vi "Main.vi"() -> ()   [LabVIEW 2020]
uses:
  controls/sliding_panel_left.ctl
  controls/power_chart.ctl
  controls/max_power_slider.ctl
  controls/tiny_map_icon_basic.ctl
  controls/sliding_panel_right.ctl
  controls/wind_chart.ctl
  controls/sliding_panel_console.ctl
  controls/day_of_month_slider.ctl
  controls/single_multicity_basic.ctl
  controls/plus_basic.ctl
  controls/minus_basic.ctl
  controls/wind_turbine_icon_basic.ctl
  controls/tiny_plots_icon_basic.ctl
  <vilib>/Platform/TimedLoop/XDataNode/timing_clust.ctl
  <vilib>/Platform/TimedLoop/XDataNode/nitl_modes.ctl
  <vilib>/Platform/TimedLoop/XDataNode/wakeup.ctl
  <vilib>/Platform/TimedLoop/XDataNode/XDataNode.xnode
  <vilib>/Platform/TimedLoop/XDataNode/XDNodeRunTimeDep.lvlib
panel:
  in  "show_map":T1
  in  "show_plots":T2
  in  "sliding_panel_console":T3={"Days of Month"=29, "multicity"=FALSE, "plus"=FALSE, "minus"=FALSE} {"Days of Month" min=1 max=30 step=1 scale=0.0..30.0}
  out "sliding_panel_right":T8={"title"="Select a city", "Wind"=[]}
  out "sliding_panel_left":T10={"title"="Power Statistics", "Power"=[], "max_power_slide"=3.1127450980392157, "max_power_digi"=0.13, "max_power_title"="Select a city (# days)"} {"max_power_digi" format="%#_3g"; "max_power_slide" scale=0.0..40.0}
  out "signature":string="Thoric 2011"
  out "title":string="Select a city"
  in  "USA":T13 caption="Texas (USA)"
  in  "costa_rica":T13 caption="Puerto Limon (Costa Rica)"
  in  "brazil":T13 caption="Brasilia (Brazil)"
  in  "south_africa":T13 caption="Cape Good Hope (South Africa)"
  in  "australia":T13 caption="Marrara (Australia)"
  in  "japan":T13 caption="Ise Bay (Japan)"
  in  "india":T13 caption="Mumbai (India)"
  in  "israel":T13 caption="Sde-Dov (Israel)"
  in  "germany":T13 caption="Berlin (Germany)"
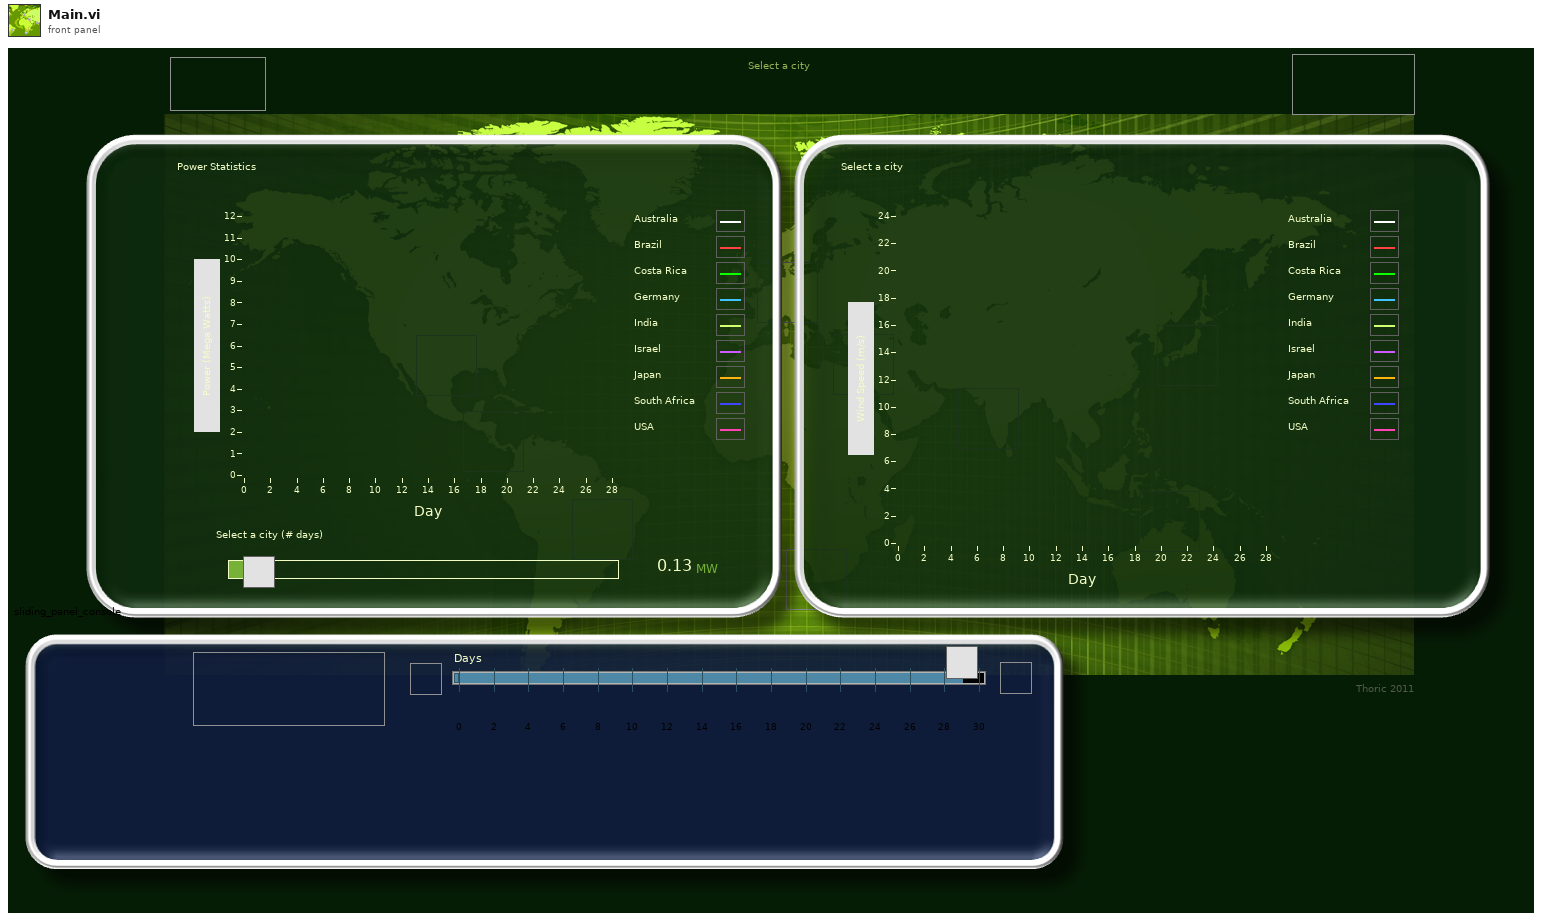
[diagram p1: front panel]
types:
  T1 = typedef "tiny_map_icon_basic.ctl" = bool
  T2 = typedef "tiny_plots_icon_basic.ctl" = bool
  T3 = typedef "sliding_panel_console.ctl" = cluster{"Days of Month":T4, "multicity":T5, "plus":T6, "minus":T7}
  T4 = typedef "day_of_month_slider.ctl" = i32
  T5 = typedef "single_multicity_basic.ctl" = bool
  T6 = typedef "plus_basic.ctl" = bool
  T7 = typedef "minus_basic.ctl" = bool
  T8 = typedef "sliding_panel_right.ctl" = cluster{"title":string, "Wind":T9}
  T9 = typedef "wind_chart.ctl" = dbl[][]
  T10 = typedef "sliding_panel_left.ctl" = cluster{"title":string, "Power":T11, "max_power_slide":T12, "max_power_digi":dbl, "max_power_title":string}
  T11 = typedef "power_chart.ctl" = dbl[][]
  T12 = typedef "max_power_slider.ctl" = dbl
  T13 = typedef "wind_turbine_icon_basic.ctl" = bool
  T14 = enum8{"Enabled", "Disabled", "Disabled and Grayed Out"}
  T15 = typedef "XDNodeRunTimeDep.lvlib/timing_clust.ctl" = cluster{"Expected End [f-1]":u64, "Actual End [f-1]":u64, "Finished Late? [f-1]":bool, "Expected End [i-1]":u64, "Actual End [i-1]":u64, "Finished Late? [i-1]":bool, "Expected Start [i]":u64, "Actual Start [i]":u64, "Expected Start [f]":u64, "Actual Start [f]":u64, "Source Name":string, "Structure Name":string, "Period":i64, "Deadline":i64, "Offset":i64, "Start":i64, "Priority":i32, "Timeout":i32, "Mode":T16, "Wakeup Reason":T17, "Error":errorcluster, "Source Type":string, "Secondary Source Type":string, "Global End Time":u64, "Global Start Time":u64, "Frame Duration":u64, "Iteration Duration":u64, "Assigned CPU":i32, "I/O Scan Engine Mode":u32}
  T16 = typedef "XDNodeRunTimeDep.lvlib/nitl_modes.ctl" = enum32{"No Change", "Process missed periods, maintain original phase", "Discard missed periods, maintain original phase", "Process missed periods, ignore original phase", "Discard missed periods, ignore original phase"}
  T17 = typedef "XDNodeRunTimeDep.lvlib/wakeup.ctl" = enum32{"Normal", "Aborted", "Asynchronous wakeup", "Timing source error", "Timed loop error", "Timeout"}
  T18 = enum32{"invalid app kind", "Development System", "Run Time System", "Student Edition", "Embedded LabVIEW", "Evaluation", "Custom"}
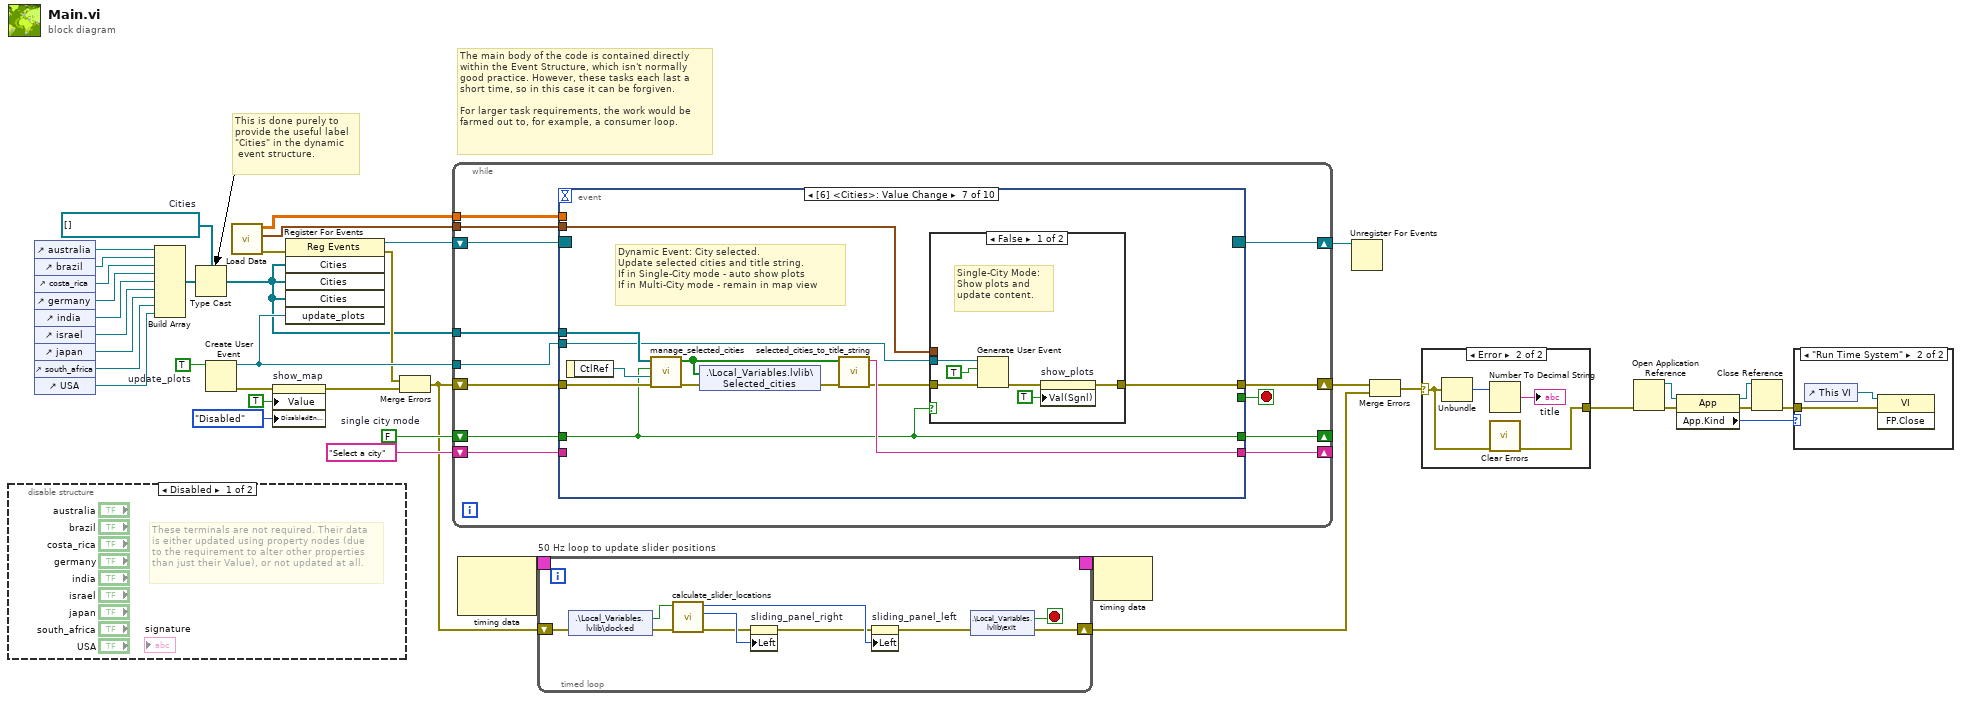
[diagram p0: block diagram]
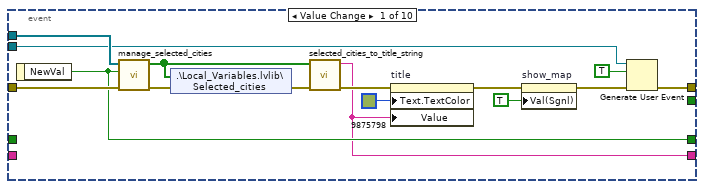
[diagram p5: hidden frame]
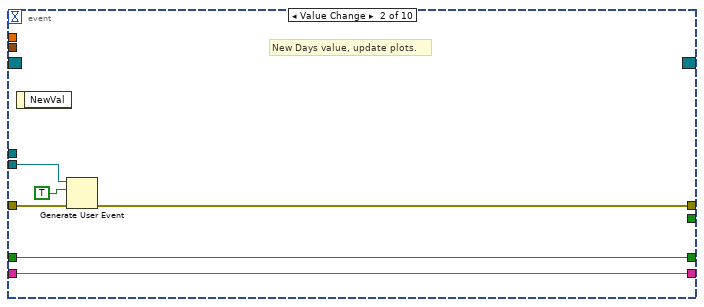
[diagram p6: hidden frame]
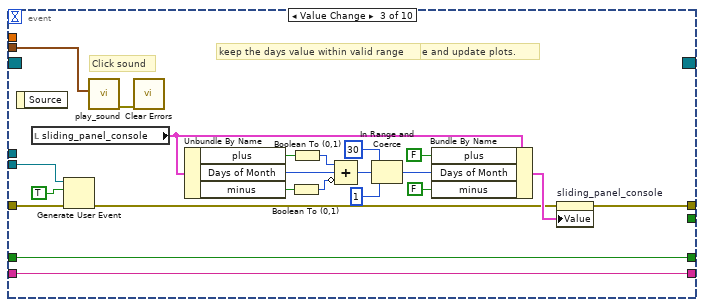
[diagram p7: hidden frame]
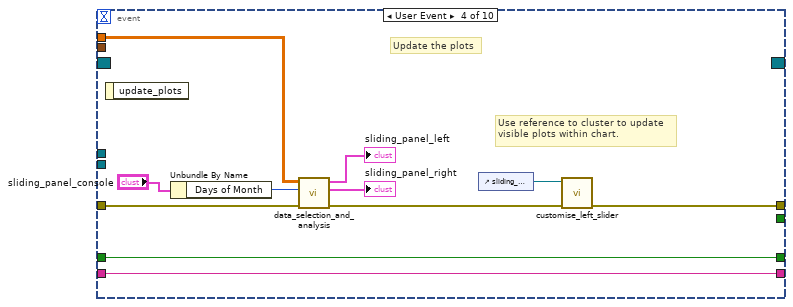
[diagram p8: hidden frame]
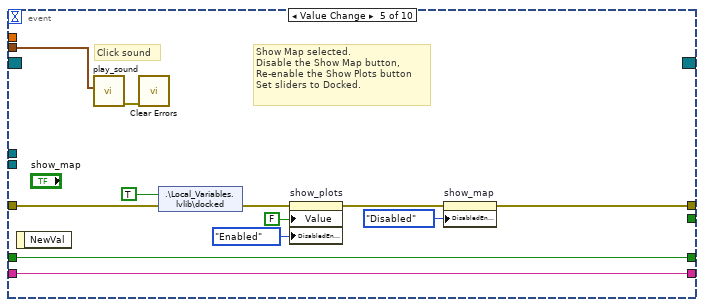
[diagram p9: hidden frame]
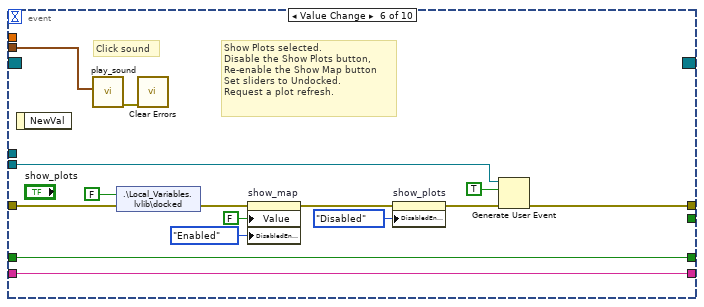
[diagram p10: hidden frame]
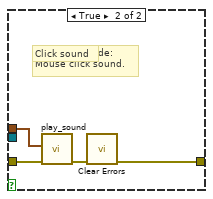
[diagram p11: hidden frame]
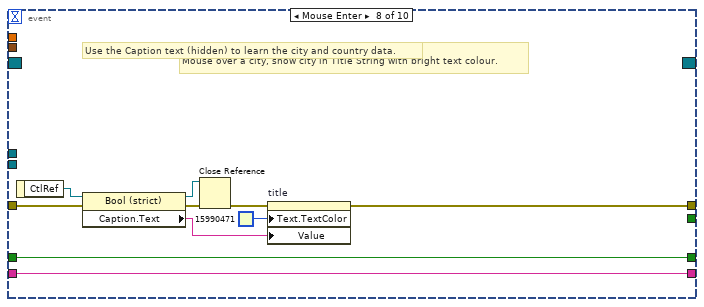
[diagram p12: hidden frame]
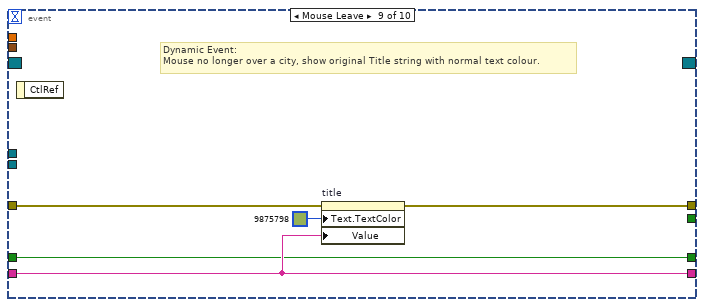
[diagram p13: hidden frame]
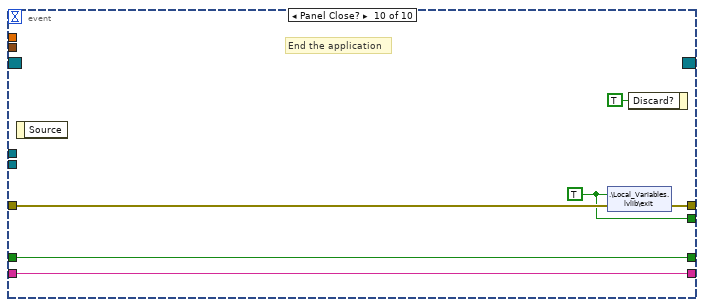
[diagram p14: hidden frame]
diagram:
  w12 = refnum<vi>[] []  # Cities
  w22 = T5 FALSE  # single city mode
  w25 = TRUE  # update_plots
  # "The main body of the code is contained directly\nwithin the Event Structure, which isn't normally\ngood practice. However, these tasks each last a\nshort time, so in this case it can be forgiven.\n\nFor larger task requirements, the work would be\nfarmed out to, for example, a consumer loop."
  # "This is done purely to\nprovide the useful label\n\"Cities\" in the dynamic\n event structure."
  n1 = disable-structure shown="Disabled" {
    frame Disabled {
      # "These terminals are not required. Their data\nis either updated using property nodes (due\nto the requirement to alter other properties\nthan just their Value), or not updated at all."
    }
    frame Enabled {
    }
  }
  n2 = control-ref of="australia"() -> (w36:refnum<vi>)
  n3 = control-ref of="brazil"() -> (w35:refnum<vi>)
  n4 = control-ref of="costa_rica"() -> (w34:refnum<vi>)
  n5 = control-ref of="germany"() -> (w33:refnum<vi>)
  n6 = control-ref of="india"() -> (w32:refnum<vi>)
  n7 = control-ref of="israel"() -> (w31:refnum<vi>)
  n8 = control-ref of="japan"() -> (w30:refnum<vi>)
  n9 = control-ref of="south_africa"() -> (w29:refnum<vi>)
  n10 = control-ref of="USA"() -> (w28:refnum<vi>)
  n11 = Build Array(w36, w35, w34, w33, w32, w31, w30, w29, w28) -> (w14:refnum<vi>[])
  n12 = Type Cast(type=w12, x=w14) -> (*(type *) &x=w13:refnum<vi>[])
  n13 = Create User Event(user event datatype=w25) -> (user event=w24:refnum<user-event>, error out=w9:errorcluster)  [unwired: 1 in]
  n14 = call "Load Data.vi"() -> ("error out"=w20:errorcluster, "Sound WAV data"=w21:waveform(dbl)[], "Wind Data"=w23:dbl[][])  [unwired: 9 in]
  n15 = property on="show_map" class="Bool (strict)"(error in=w9, "Value"=TRUE, "DisabledEnum"=T14."Disabled" ("Disabled")) -> (error out=w8:errorcluster)  [unwired: 1 in, 1 out]
  n16 = register-events(error in=w20, w13, w13, w13, w24) -> (reference out=w37:refnum<event-registration>, error out=w19:errorcluster)  [unwired: 1 in]
  n17 = Merge Errors(w19, w8) -> (w18:errorcluster)
  n18 = while {
    shift-right: [w51] -> w17
    shift-left: w18 -> [w52]
    shift-right: [w48] -> w27
    shift-left: w37 -> [w49]
    shift-right: [w46] -> _
    shift-left: "Select a city" ("title") -> [w47]
    shift-right: [w44] -> _
    shift-left: w22 -> [w45]
    tunnel: w13 -> [w43]
    tunnel: w24 -> [w42]
    tunnel: w23 -> [w41]
    tunnel: w21 -> [w40]
    stop <- w50 stop-if-true
    n19 = event shown="[6] <Cities>: Value Change" {
      selector: w49 -> [_ _ _ _ _ _ _ _ _ _]
      dyn-events: [_ _ _ _ _ _ _ _ _ _] -> w48
      timeout: _ -> [_ _ _ _ _ _ _ _ _ _]
      tunnel: w52 -> [w67 w70 w81 w104 w116 w131 w141 w159 w169 w175]
      tunnel: [w55 w68 w93 w96 w110 w128 w136 w163 w168 w176] -> w51
      tunnel: [_ _ _ _ _ _ _ _ _ w174] -> w50
      tunnel: w47 -> [_ w73 w95 w106 w118 w133 _ w164 w167 w172]
      tunnel: [w59 w73 w95 w106 w118 w133 w144 w164 w167 w172] -> w46
      tunnel: w45 -> [_ w72 w94 w105 w117 w132 w138 w160 w166 w171]
      tunnel: [w66 w72 w94 w105 w117 w132 w138 w160 w166 w171] -> w44
      tunnel: w43 -> [w65 _ _ _ _ _ w143 _ _ _]
      tunnel: w42 -> [w54 w69 w79 _ _ w124 w134 _ _ _]
      tunnel: w41 -> [_ _ _ w103 _ _ _ _ _ _]
      tunnel: w40 -> [_ _ w74 _ w107 w119 w135 _ _ _]
      event Value Change {
        n20 = event-data() -> ("NewVal"=w66:T5)  [unwired: 1 in]
        n21 = call "manage_selected_cities.vi"("error in"=w67, "multicity"=w66, "Selected_cities_refs[]"=w65) -> ("error out"=w64:errorcluster, "Selected_Cities[]"=w62:T13[])  [unwired: 7 in]
        n22 = shared-variable ".\\Local_Variables.lvlib\\Selected_cities"(w62, error in=w64) -> (error out=w63:errorcluster)
        n23 = call "selected_cities_to_title_string.vi"("error in"=w63, "selected_cities"=w62) -> ("error out"=w60:errorcluster, "title_string"=w59:string)  [unwired: 8 in]
        n24 = property on="title" class="Str"(error in=w60, "Text.TextColor"=u32 9875798, "Value"=w59) -> (error out=w58:errorcluster)  [unwired: 1 in, 1 out]
        n25 = property on="show_map" class="Bool (strict)"(error in=w58, "Val(Sgnl)"=TRUE ("docked")) -> (error out=w56:errorcluster)  [unwired: 1 in, 1 out]
        n26 = Generate User Event(user event=w54, event data cluster=TRUE ("event data"), error in=w56) -> (error out=w55:errorcluster)  [unwired: 1 in, 1 out]
      }
      event Value Change {
        # "New Days value, update plots."
        n27 = event-data() -> ()  [unwired: 1 in, 1 out]
        n28 = Generate User Event(user event=w69, event data cluster=TRUE ("event data"), error in=w70) -> (error out=w68:errorcluster)  [unwired: 1 in, 1 out]
      }
      event Value Change {
        # "keep the days value within valid range"
        # "Days +, Days - selected. Update Days value and update plots."
        # "Click sound"
        n29 = event-data() -> ()  [unwired: 1 in, 1 out]
        n30 = local read "sliding_panel_console"() -> (w92:T3)
        n31 = Generate User Event(user event=w79, event data cluster=TRUE ("event data"), error in=w81) -> (error out=w80:errorcluster)  [unwired: 1 in, 1 out]
        n32 = call "play_sound.vi"("Data"=w74) -> ("error out"=w75:errorcluster)  [unwired: 9 in]
        n33 = call <vilib>:"Clear Errors.vi"("error in (no error)"=w75) -> ()  [unwired: 5 in, 2 out]
        n34 = Unbundle By Name(w92) -> ("plus"=w88:T6, "Days of Month"=w89:T4, "minus"=w86:T7)
        n35 = Boolean To (0,1)(Boolean=w86) -> (0, 1=w85:i16)
        n36 = Boolean To (0,1)(Boolean=w88) -> (0, 1=w87:i16)
        n37 = Compound Arithmetic op=ADD(w87, w89, invert w85) -> (w90:T4)
        n38 = In Range and Coerce(upper limit=T4 30, x=w90, lower limit=T4 1) -> (coerced(x)=w78:T4)  [unwired: 1 out]
        n39 = Bundle By Name(cluster=w92, "plus"=T6 FALSE, "Days of Month"=w78, "minus"=T7 FALSE) -> (w91:T3)
        n40 = property on="sliding_panel_console" class="Clust (strict)"(error in=w80, "Value"=w91) -> (error out=w93:errorcluster)  [unwired: 1 in, 1 out]
      }
      event User Event {
        # "Use reference to cluster to update\nvisible plots within chart."
        # "Update the plots"
        n41 = event-data() -> ()  [unwired: 1 in, 1 out]
        n42 = Unbundle By Name("sliding_panel_console") -> ("Days of Month"=w101:T4)
        n43 = call "data_selection_and_analysis.vi"("error in"=w104, "days"=w101, "wind data in"=w103) -> ("error out"=w97:errorcluster, "sliding_panel_right"=→"sliding_panel_right":T8, "left_pane_cluster"=→"sliding_panel_left":T10)  [unwired: 6 in]
        n44 = control-ref of="sliding_panel_left"() -> (w98:refnum<vi>)
        n45 = call "customise_left_slider.vi"("error in"=w97, "slide_left_ref"=w98) -> ("error out"=w96:errorcluster)  [unwired: 9 in]
      }
      event Value Change {
        # "Show Map selected.\nDisable the Show Map button,\nRe-enable the Show Plots button\nSet sliders to Docked."
        # "Click sound"
        n46 = event-data() -> ()  [unwired: 1 in, 1 out]
        n47 = call "play_sound.vi"("Data"=w107) -> ("error out"=w108:errorcluster)  [unwired: 9 in]
        n48 = call <vilib>:"Clear Errors.vi"("error in (no error)"=w108) -> ()  [unwired: 5 in, 2 out]
        n49 = shared-variable ".\\Local_Variables.lvlib\\docked"(TRUE, error in=w116) -> (error out=w114:errorcluster)
        n50 = property on="show_plots" class="Bool (strict)"(error in=w114, "Value"=FALSE ("hide_map"), "DisabledEnum"=T14."Enabled" ("Disabled")) -> (error out=w111:errorcluster)  [unwired: 1 in, 1 out]
        n51 = property on="show_map" class="Bool (strict)"(error in=w111, "DisabledEnum"=T14."Disabled" ("Disabled")) -> (error out=w110:errorcluster)  [unwired: 1 in, 1 out]
      }
      event Value Change {
        # "Show Plots selected.\nDisable the Show Plots button,\nRe-enable the Show Map button\nSet sliders to Undocked.\nRequest a plot refresh."
        # "Click sound"
        n52 = event-data() -> ()  [unwired: 1 in, 1 out]
        n53 = call "play_sound.vi"("Data"=w119) -> ("error out"=w120:errorcluster)  [unwired: 9 in]
        n54 = shared-variable ".\\Local_Variables.lvlib\\docked"(FALSE, error in=w131) -> (error out=w127:errorcluster)
        n55 = call <vilib>:"Clear Errors.vi"("error in (no error)"=w120) -> ()  [unwired: 5 in, 2 out]
        n56 = property on="show_map" class="Bool (strict)"(error in=w127, "Value"=FALSE, "DisabledEnum"=T14."Enabled" ("Disabled")) -> (error out=w123:errorcluster)  [unwired: 1 in, 1 out]
        n57 = property on="show_plots" class="Bool (strict)"(error in=w123, "DisabledEnum"=T14."Disabled" ("Disabled")) -> (error out=w122:errorcluster)  [unwired: 1 in, 1 out]
        n58 = Generate User Event(user event=w124, event data cluster=TRUE ("event data"), error in=w122) -> (error out=w128:errorcluster)  [unwired: 1 in, 1 out]
      }
      event Value Change {
        # "Dynamic Event: City selected.\nUpdate selected cities and title string.\nIf in Single-City mode - auto show plots\nIf in Multi-City mode - remain in map view"
        n59 = event-data() -> ("CtlRef"=w139:refnum<vi>)  [unwired: 1 in]
        n60 = call "manage_selected_cities.vi"("error in"=w141, "selected_city"=w139, "multicity"=w138, "Selected_cities_refs[]"=w143) -> ("error out"=w140:errorcluster, "Selected_Cities[]"=w142:T13[])  [unwired: 6 in]
        n61 = shared-variable ".\\Local_Variables.lvlib\\Selected_cities"(w142, error in=w140) -> (error out=w145:errorcluster)
        n62 = call "selected_cities_to_title_string.vi"("error in"=w145, "selected_cities"=w142) -> ("error out"=w137:errorcluster, "title_string"=w144:string)  [unwired: 8 in]
        n63 = case shown="False" w138 {
          tunnel: w137 -> [w147 w153]
          tunnel: [w150 w152] -> w136
          tunnel: w134 -> [w148 _]
          tunnel: w135 -> [_ w154]
          frame False {
            # "Single-City Mode:\nShow plots and\nupdate content."
            n64 = Generate User Event(user event=w148, event data cluster=TRUE ("event data"), error in=w147) -> (error out=w146:errorcluster)  [unwired: 1 in, 1 out]
            n65 = property on="show_plots" class="Bool (strict)"(error in=w146, "Val(Sgnl)"=TRUE ("docked")) -> (error out=w150:errorcluster)  [unwired: 1 in, 1 out]
          }
          frame True {
            # "Multi-City mode:\nMouse click sound."
            # "Click sound"
            n66 = call "play_sound.vi"("error in"=w153, "Data"=w154) -> ("error out"=w155:errorcluster)  [unwired: 8 in]
            n67 = call <vilib>:"Clear Errors.vi"("error in (no error)"=w155) -> ("error out"=w152:errorcluster)  [unwired: 5 in, 1 out]
          }
        }
      }
      event Mouse Enter {
        # "Use the Caption text (hidden) to learn the city and country data."
        # "Dynamic Event:\nMouse over a city, show city in Title String with bright text colour."
        n68 = event-data() -> ("CtlRef"=w165:refnum<vi>)  [unwired: 1 in]
        n69 = property class="Bool (strict)"(reference=w165, error in=w159) -> (reference out=w157:refnum<vi>, error out=w158:errorcluster, "Caption.Text"=w161:string)
        n70 = Close Reference(reference=w157, error in (no error)=w158) -> (error out=w156:errorcluster)
        n71 = property on="title" class="Str"(error in=w156, "Text.TextColor"=u32 15990471, "Value"=w161) -> (error out=w163:errorcluster)  [unwired: 1 in, 1 out]
      }
      event Mouse Leave {
        # "Dynamic Event:\nMouse no longer over a city, show original Title string with normal text colour."
        n72 = event-data() -> ()  [unwired: 1 in, 1 out]
        n73 = property on="title" class="Str"(error in=w169, "Text.TextColor"=u32 9875798, "Value"=w167) -> (error out=w168:errorcluster)  [unwired: 1 in, 1 out]
      }
      event Panel Close? {
        w174 = TRUE ("exit")
        # "End the application"
        n74 = event-data() -> ()  [unwired: 1 in, 1 out]
        n75 = shared-variable ".\\Local_Variables.lvlib\\exit"(w174, error in=w175) -> (error out=w176:errorcluster)
        n76 = event-data("Discard?"=TRUE) -> ()  [unwired: 1 in, 1 out]
      }
    }
  }
  n77 = node-c288() -> (w39:T15)  [unwired: 2 in]
  n78 = timed-loop "50 Hz loop to update slider positions" {
    timing: w39 -> [_]
    timing-out: [_] -> w38
    shift-right: [w177] -> w16
    shift-left: w18 -> [w178]
    stop <- w183 stop-if-true
    n79 = shared-variable ".\\Local_Variables.lvlib\\docked"(error in=w178) -> (w184:bool, error out=w182:errorcluster)
    n80 = call "calculate_slider_locations.vi"("error in"=w182, "Docked? (F)"=w184) -> ("error out"=w181:errorcluster, "sliding_panel_right_coord"=w185:i32, "sliding_panel_left_coord"=w186:i32)  [unwired: 7 in]
    n81 = property on="sliding_panel_right" class="Clust (strict)"(error in=w181, "Left"=w185) -> (error out=w180:errorcluster)  [unwired: 1 in, 1 out]
    n82 = property on="sliding_panel_left" class="Clust (strict)"(error in=w180, "Left"=w186) -> (error out=w179:errorcluster)  [unwired: 1 in, 1 out]
    n83 = shared-variable ".\\Local_Variables.lvlib\\exit"(error in=w179) -> (w183:bool, error out=w177:errorcluster)
  }
  n84 = node-c288(w38) -> ()  [unwired: 1 out]
  n85 = Unregister For Events(event registration refnum=w27) -> ()  [unwired: 1 in, 1 out]
  n86 = Merge Errors(w17, w16) -> (w15:errorcluster)
  n87 = case shown="Error" w15 {
    selector: w15 -> [w189 w191]
    tunnel: [w189 w190] -> w2
    frame No Error {
    }
    frame Error {
      n88 = Unbundle(w191) -> ("code"=w193:i32)  [unwired: 2 out]
      n89 = Number To Decimal String(number=w193) -> (decimal integer string=→"title":string)  [unwired: 1 in]
      n90 = call <vilib>:"Clear Errors.vi"("error in (no error)"=w191) -> ("error out"=w190:errorcluster)  [unwired: 5 in, 1 out]
    }
  }
  n91 = Open Application Reference(8:w2) -> (0:w6:errorcluster, 3:w7:refnum<vi>)  [unwired: 3 in]
  n92 = property class="App"(reference=w7, error in=w6) -> (reference out=w4:refnum<vi>, error out=w5:errorcluster, "App.Kind"=w3:T18)
  n93 = Close Reference(reference=w4, error in (no error)=w5) -> (error out=w1:errorcluster)
  n94 = case shown="\"Run Time System\"" w3 {
    tunnel: w1 -> [_ w194]
    frame "Development System", Default {
    }
    frame "Run Time System" {
      n95 = control-ref of="This VI"() -> (w195:refnum<vi>)
      n96 = invoke class="VI" method="FP.Close"(reference=w195, error in=w194) -> ()  [unwired: 1 in, 3 out]
    }
  }
